vi "Write GUID.vi"(8 "error in (no error)":errorcluster, 10 "GUID":string, 11 "Client Controller in":refnum<class "Client Controller.lvclass">) -> (0 "error out":errorcluster, 3 "Client Controller out":refnum<class "Client Controller.lvclass">)   [LabVIEW 2026, in "Client Controller.lvlib" / "Client Controller.lvclass"]
uses:
  Client Controller.lvclass
  Client Controller.lvclass/Client Controller.ctl
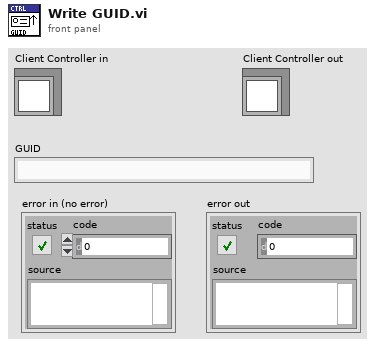
[diagram p1: front panel]
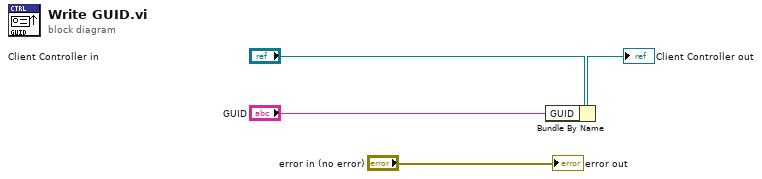
[diagram p0: block diagram]
diagram:
  n1 = Bundle By Name(cluster="Client Controller in", "GUID"="GUID") -> (→"Client Controller out":refnum<class "Client Controller.lvclass">)
  "error out" <- "error in (no error)"
